vi "TreeViewRestoreState.vi"(8 "error in (no error)":errorcluster, 10 "State":T1, 11 "TreeControl in":refnum<vi>) -> (0 "error out":errorcluster, 3 "TreeControl out":refnum<vi>)   [LabVIEW 2021, in "VIPropertyPicker.lvlib"]
uses:
  VIPropertyPicker.lvlib
  <vilib>/Utility/Data Type/NI_Data Type.lvlib
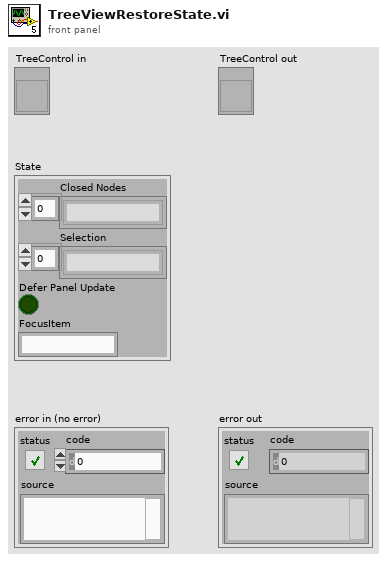
[diagram p1: front panel]
types:
  T1 = cluster{"Closed Nodes":string[], "Selection":string[], "Defer Panel Update":bool, "FocusItem":string}
  T2 = typedef "NI_Data Type.lvlib/Data Type.ctl" = enum8{"Invalid Type", "Void", "I8", "I16", "I32", "I64", "U8", "U16", "U32", "U64", "Single Float", "Double Float", "Extended Float", "Single Complex", "Double Complex", "Extended Complex", "Enum U8", "Enum U16", "Enum U32", "Enum U64", "Single Float With Unit", "Double Float With Unit", "Extended Float With Unit", "Single Complex with Unit", "Double Complex with Unit", "Extended Complex with Unit", "Boolean", "String", "Path", "Picture", "Tag", "Array", "Cluster", "Variant", "LV Variant", "Waveform", "Timestamp", "Digital Waveform", "Digital Data", "ExpressData", "Refnum", "External Data", "VI", "Poly VI", "LabVIEW Class Instance", "Fixed Point", "Set Collection", "Map Collection"}
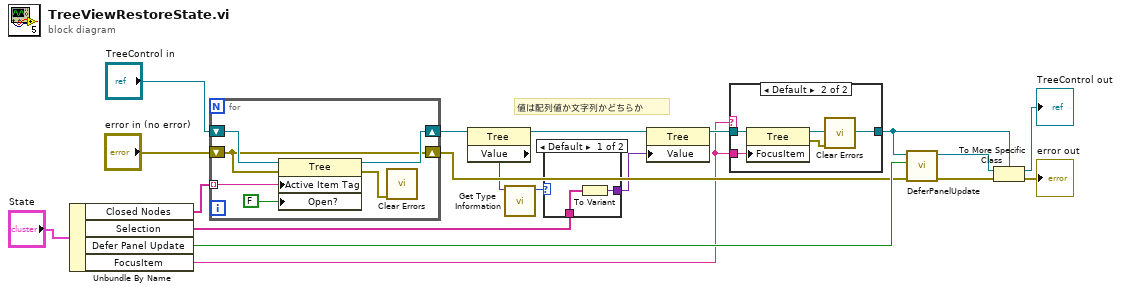
[diagram p0: block diagram]
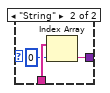
[diagram p3: hidden frame]
diagram:
  # "値は配列値か文字列かどちらか"
  n1 = Unbundle By Name("State") -> ("Closed Nodes"=w17:string[], "Selection"=w5:string[], "Defer Panel Update"=w11:bool, "FocusItem"=w1:string)
  n2 = for {
    tunnel: w17 -> [w24] mode=indexing
    shift-right: [w22] -> w10
    shift-left: "TreeControl in" -> [w23]
    shift-right: [w21] -> w9
    shift-left: "error in (no error)" -> [w21]
    n3 = property class="Tree"(reference=w23, error in=w21, "Active Item Tag"=w24, "Open?"=FALSE ("Active Item:Open?")) -> (reference out=w22:refnum<vi>, error out=w20:errorcluster)
    n4 = call <vilib>:"Clear Errors.vi"("error in (no error)"=w20) -> ()  [unwired: 5 in, 2 out]
  }
  n5 = property class="Tree"(reference=w10) -> (reference out=w8:refnum<vi>, "Value"=w7:variant)  [unwired: 1 in, 1 out]
  n6 = call <vilib>:"Get Type Information.vi"("variant"=w7) -> ("type"=w6:T2)  [unwired: 6 in, 4 out]
  n7 = case shown="Default" w6 {
    tunnel: w5 -> [w26 w30]
    tunnel: [w27 w28] -> w4
    frame Default {
      n8 = To Variant(anything=w26) -> (Variant=w27:variant)
    }
    frame "String" {
      n9 = Index Array(array=w30, index=0) -> (element=w28:string)
    }
  }
  n10 = property class="Tree"(reference=w8, "Value"=w4) -> (reference out=w14:refnum<vi>)  [unwired: 1 in, 1 out]
  n11 = case shown="Default" w1 {
    tunnel: w14 -> [w31 w35]
    tunnel: [w31 w34] -> w2
    tunnel: w1 -> [_ w33]
    frame "" {
    }
    frame Default {
      n12 = property class="Tree"(reference=w35, "FocusItem"=w33) -> (reference out=w34:refnum<vi>, error out=w32:errorcluster)  [unwired: 1 in]
      n13 = call <vilib>:"Clear Errors.vi"("error in (no error)"=w32) -> ()  [unwired: 5 in, 2 out]
    }
  }
  n14 = call "DeferPanelUpdate.vi"("error in (no error)"=w9, "Defer Panel Updates (T)"=w11, "Control in"=w2) -> ("error out"=w15:errorcluster, "Control out"=w12:refnum<vi>)  [unwired: 6 in, 1 out]
  n15 = To More Specific Class(target class=w2, reference=w12, error in=w15) -> (specific class reference=→"TreeControl out":refnum<vi>, error out=→"error out":errorcluster)
